vi "Logger.Begin.vi"(8 "error in":errorcluster, 10 "Data in":T1={"BeginTS"=timestamp(0 s since 1904-01-01), "EndTS"=timestamp(0 s since 1904-01-01), "State"=enum."Init", "Status.Work"=enum."-", "Status.Process"=enum."-", "Status.Home"=enum."-", "Status.Wabco"=enum."-", "Status.Client"=enum."-", "BreakReason"=enum."-", "BreakSource"=enum."-", "DoorLock"=FALSE, "Status.Prod"=[], "UserAction"={"Stop"=FALSE, "Pause"=FALSE, "Next"=FALSE}, "UserData"={"GuiMode"=enum."Process", "Test"={"IgnoreResults"=FALSE, "IgnoreImages"=FALSE, "ServiceMode"=FALSE}, "ContinueOrder"=FALSE}, "Error"={"status"=FALSE, "code"=0, "source"=""}, "Code"={"Ready"=FALSE, "DoubleOrder"=FALSE, "OrderDone"=FALSE, "AllowSingleSlot"=FALSE, "CheckDM"=FALSE, "ThresholdA"=0, "ThresholdB"=0, "Plate"=enum."Wabco", "ImgPath"=path "", "Variant"={"State"=enum."Init", "ImgPath"=path "", "WabcoPlate"="", "WabcoProduct"="", "ClientProduct"="", "ClientPlate"="", "TotalQuantity"=0, "OrderQuantity"=0, "Serial"=0, "Wabco"={"LaserJob"="", "AdditionalTxt"="037", "FactoryCode"="", "RevID"=0, "ForkID"=0, "FailuresLimit"=0, "GlobalCnt"=0, "ScannerProgram"=0, "SerialFormat"=enum."6 dig", "CoordA"={"X"=0.0, "Y"=0.0, "Angle"=0.0}, "CoordB"={"X"=0.0, "Y"=0.0, "Angle"=0.0}, "DMCconfig"=0}, "Client"={"LaserJob"="", "AdditionalTxt"="", "FactoryCode"="037", "RevID"=0, "ForkID"=0, "FailuresLimit"=0, "GlobalCnt"=0, "ScannerProgram"=0, "SerialFormat"=enum."6 dig", "CoordA"={"X"=0.0, "Y"=0.0, "Angle"=0.0}, "CoordB"={"X"=0.0, "Y"=0.0, "Angle"=0.0}, "DMCconfig"=0}}}, "Rotations"=0, "ProdIdx"=0, "ProdDone"=[], "PrintedSerials-Wabco"=[], "PrintedSerials-Client"=[], "Counters-Wabco"={"Expected"=0, "Done"=0, "OK"=0, "NOK"=0, "NOKlimit"=0, "Part"=0, "PartOK"=0}, "Counters-Client"={"Expected"=0, "Done"=0, "OK"=0, "NOK"=0, "NOKlimit"=0, "Part"=0, "PartOK"=0}}) -> (0 "error out":errorcluster, 2 "Folder":path, 3 "Refnum out":refnum<k34>)   [LabVIEW 2016]
uses:
  tools/Translator/Translator.Message.ctl
  tools/EventLog/EventLog.EventSource.ctl
  Global/ApplicationGlobal.vi
  tools/EventLog/EventLog.New(single).vi
  Sequence/Sequence.State.ctl
  Gui/MainGui.TestOptions.ctl
  Sequence/Sequence.MainMode.ctl
  Sequence/Sequence.UserData.ctl
  Sequence/Sequence.UserActions.ctl
  Sequence/Sequence.Step.Status.ctl
  Sequence/Sequence.Test.BreakReason.ctl
  Sequence/Sequence.Prod.StatusData.ctl
  Sequence/Sequence.Test.Unload.Status.ctl
  Sequence/Sequence.Slot.StatusData.ctl
  Sequence/Sequence.Test.Status.ctl
  Sequence/Sequence.Code.Sets.ctl
  Sequence/Sequence.Data.ctl
  Logger.Variant.Sets.ctl
  Station/Station.Changeover.State.vi
  Sequence/Sequence.Code.SerialFormat.ctl
  Station/Station.Plate.Properties.ctl
  Drivers/V7310/LowLevel/V7310.Job.Sets.ctl
  Sequence/Sequence.PlateType.ctl
  Sequence/Sequence.Counters.ctl
  Sequence/Sequence.Test.BreakSource.ctl
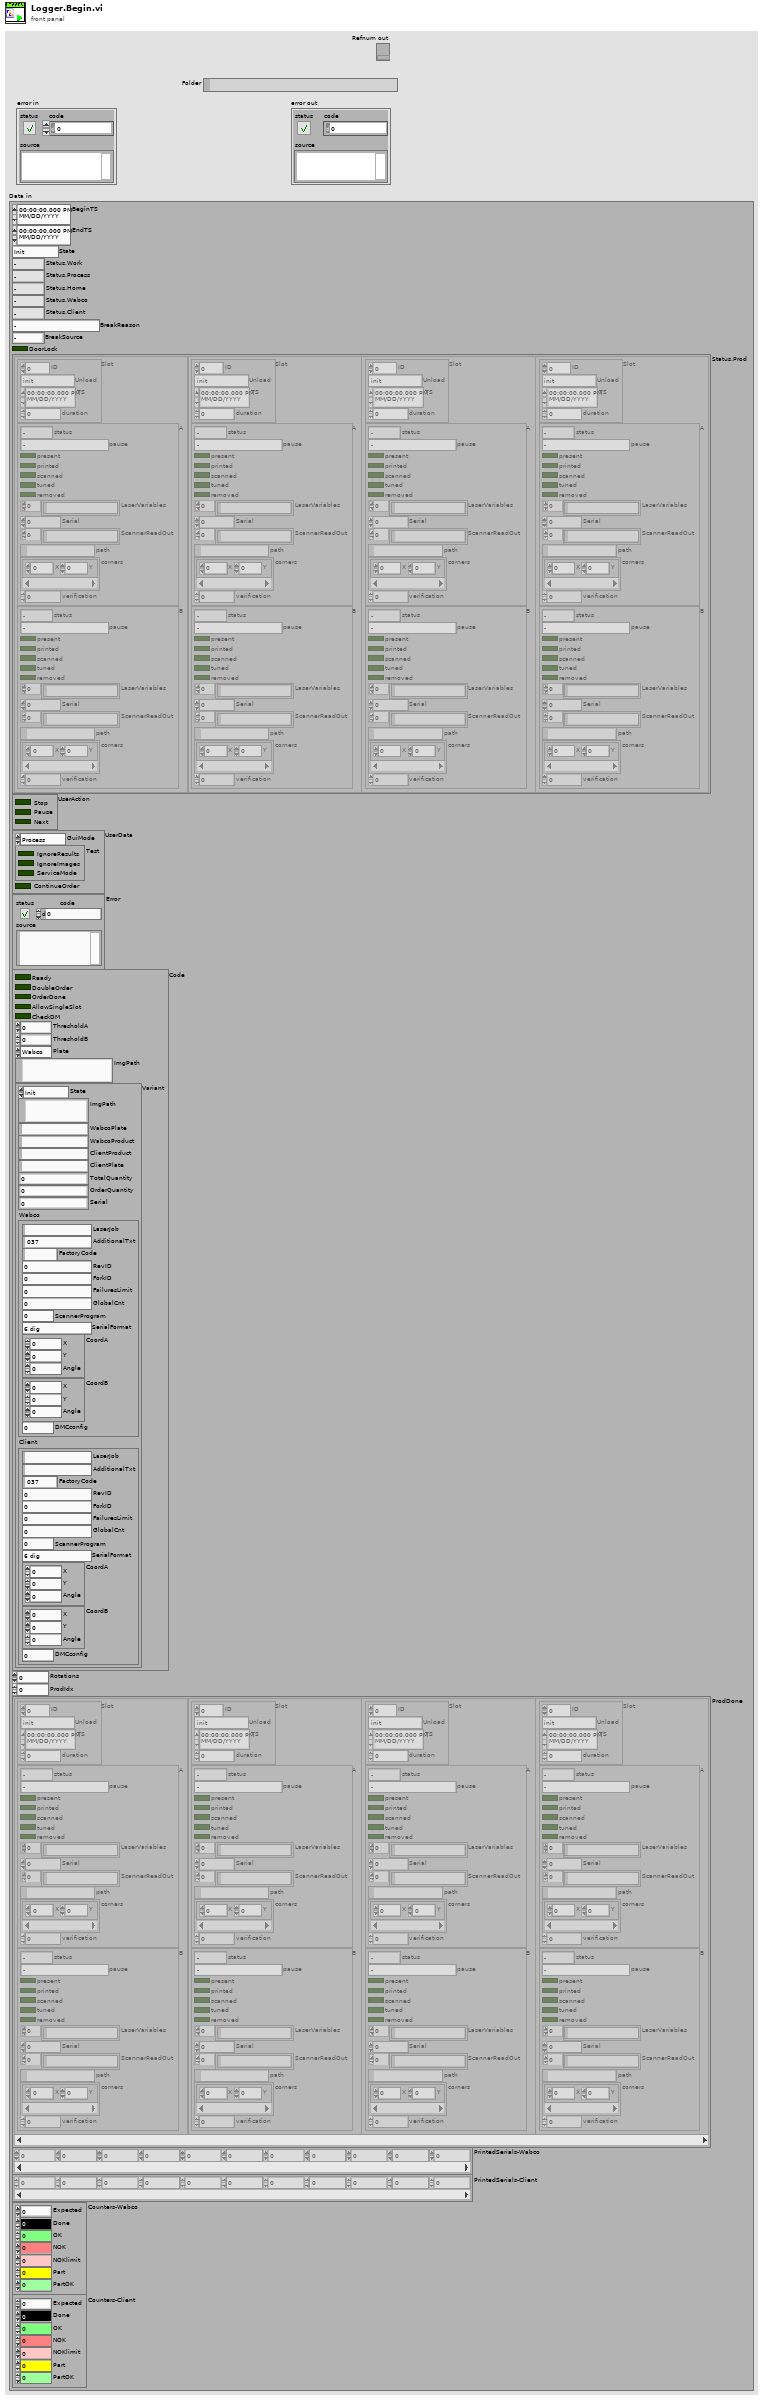
[diagram p1: front panel]
types:
  T1 = typedef "Sequence.Data.ctl" = cluster{"BeginTS":timestamp, "EndTS":timestamp, "State":T2, "Status.Work":T3, "Status.Process":T3, "Status.Home":T3, "Status.Wabco":T3, "Status.Client":T3, "BreakReason":T4, "BreakSource":T5, "DoorLock":bool, "Status.Prod":T6[], "UserAction":T10, "UserData":T11, "Error":errorcluster, "Code":T14, "Rotations":i32, "ProdIdx":i32, "ProdDone":T6[], "PrintedSerials-Wabco":i32[], "PrintedSerials-Client":i32[], "Counters-Wabco":T21, "Counters-Client":T21}
  T2 = typedef "Sequence.State.ctl" = enum16{"Init", "Idle", "Home", "Work", "Run", "Pause"}
  T3 = typedef "Sequence.Step.Status.ctl" = enum16{"-", "Pending", "Running", "Skipped", "Passed", "Failed", "Done", "Error", "Aborted", "Stopped"}
  T4 = typedef "Sequence.Test.BreakReason.ctl" = enum16{"-", "NOK container", "OK container", "Rev empty", "Rev missing", "Rev wrong", "Fork missing", "Fork wrong", "NOK limit", "Unload failure", "Single slot", "Part done", "Err: Prod move work", "Err: Prod move home", "Err: Prod lift work", "Err: Prod lift home", "Err: Prod Arm Work", "Err: Prod Arm NOK", "Err: Prod Arm OK", "Err: Prod NOK suck", "Err: Prod NOK drop", "Err: Prod OK missing", "Err: Prod OK suck", "Err: Prod OK drop"}
  T5 = typedef "Sequence.Test.BreakSource.ctl" = enum16{"-", "A", "B", "A/B"}
  T6 = typedef "Sequence.Test.Status.ctl" = cluster{"Slot":T7, "A":T9, "B":T9}
  T7 = typedef "Sequence.Slot.StatusData.ctl" = cluster{"ID":i32, "Unload":T8, "TS":timestamp, "duration":u32}
  T8 = typedef "Sequence.Test.Unload.Status.ctl" = enum16{"init", "check NOK", "check OK", "wait on NOK", "wait on OK", "wait on Unload", "done"}
  T9 = typedef "Sequence.Prod.StatusData.ctl" = cluster{"status":T3, "pause":T4, "present":bool, "printed":bool, "scanned":bool, "tuned":bool, "removed":bool, "LaserVariables":string[], "Serial":i32, "ScannerReadOut":string[], "path":path, "corners":cluster{"X":i32, "Y":i32}[], "verification":u8}
  T10 = typedef "Sequence.UserActions.ctl" = cluster{"Stop":bool, "Pause":bool, "Next":bool}
  T11 = typedef "Sequence.UserData.ctl" = cluster{"GuiMode":T12, "Test":T13, "ContinueOrder":bool}
  T12 = typedef "Sequence.MainMode.ctl" = enum16{"Process", "Base", "Order", "Manual", "Logs", "Results", "Stats", "DMC Config"}
  T13 = typedef "MainGui.TestOptions.ctl" = cluster{"IgnoreResults":bool, "IgnoreImages":bool, "ServiceMode":bool}
  T14 = typedef "Sequence.Code.Sets.ctl" = cluster{"Ready":bool, "DoubleOrder":bool, "OrderDone":bool, "AllowSingleSlot":bool, "CheckDM":bool, "ThresholdA":u8, "ThresholdB":u8, "Plate":T15, "ImgPath":path, "Variant":T16}
  T15 = typedef "Sequence.PlateType.ctl" = enum16{"Wabco", "Client"}
  T16 = typedef "Logger.Variant.Sets.ctl" = cluster{"State":T17, "ImgPath":path, "WabcoPlate":string, "WabcoProduct":string, "ClientProduct":string, "ClientPlate":string, "TotalQuantity":u16, "OrderQuantity":u16, "Serial":i32, "Wabco":T18, "Client":T18}
  T17 = typedef "Station.Changeover.State.vi" = enum16{"Init", "Scaning", "NOK", "Wait for ack", "Ready"}
  T18 = typedef "Station.Plate.Properties.ctl" = cluster{"LaserJob":string, "AdditionalTxt":string, "FactoryCode":string, "RevID":u8, "ForkID":u8, "FailuresLimit":u16, "GlobalCnt":i32, "ScannerProgram":u8, "SerialFormat":T19, "CoordA":T20, "CoordB":T20, "DMCconfig":i32}
  T19 = typedef "Sequence.Code.SerialFormat.ctl" = enum8{"", "6 dig", "7 dig"}
  T20 = typedef "V7310.Job.Sets.ctl" = cluster{"X":dbl, "Y":dbl, "Angle":dbl}
  T21 = typedef "Sequence.Counters.ctl" = cluster{"Expected":u16, "Done":u16, "OK":u16, "NOK":u16, "NOKlimit":u16, "Part":u16, "PartOK":u16}
  T22 = typedef "EventLog.EventSource.ctl" = enum16{"All", "Gui", "Ref", "File", "Arch", "Seq", "CPX", "DB", "Laser", "Scan.P", "Scan.O"}
  T23 = typedef "Translator.Message.ctl" = enum16{"-", "Event confirmed", "Log out", "Log in", "Shutdown", "Cancel", "Start", "Begin time", "End time", "Duration", "Service Mode", "Ignore Results", "Serial Format", "On", "Off", "OK", "NOK", "NOK %s", "Home", "Work", "Close", "Open", "In progress...", "Missing", "Empty", "Hardware failure", "Initial", "Default", "Total", "Out of range", "Free disk space is below 1GB - contact technician", "Error %d >> %s", "Error %d >> %s >> %s", "Msg %d >> %s", "Laser msg %d %s", "Laser cmd error %s %d", "Laser cmd failed %s", "Laser cmd warning %s", "Laser disconnected", "Laser status %s", "Laser already started", "Laser job unkonwn %s", "Laser job missing %s", "Laser job select failure %s", "Unable to start laser printing (%s)", "Unable to stop laser printing (%s)", "Laser marking aborted", "Laser marking timeout", "Unable to reset Laser Interlock (%s)", "Unable to trigger Laser. Laser not ready (%s)", "Laser job '%s' coordinates not configured", "Starting %s", "Quitting %s", "Configured", "Initializing", "Quitting", "Loading", "Loaded %d results", "Loaded %d events", "Running", "Stopped", "Summary", "Laser", "Do you want to continue?", "Do you want to delete the configuration?", "The configuration is being used by an order. Unable to delete!", "Press confirm button", "Station is not based. Do you want to exit?", "Station requires changeover. Do you want to run the test?", "Test options are not set as default. Do you want to continue?", "Formatting of WabcoNo is disabled. Do you want to continue?", "Product not detected. Do you want to continue?", "Product scan failed. Do you want to continue?", "Calibration", "Log out?", "System", "All", "IDLE", "Translating...%s", "Not found", "Alarm %s", "Run", "Skip", "Abort", "Repeat", "Please wait...", "Database disconnected", "Database disconnected - changeover disabled!", "Login to database successful", "Login to database failed: %d; %s", "Unable to check the product status of reference %d - database disconnected", "Unable to set the product status of reference %d - database disconnected", "Variant file backup %s", "Read variant (%s)", "Result", "Station armed!", "Station requires changeover!", "Select reference number...", "EMERGENCY BUTTON - press Control button", "EMERGENCY DOOR - press Control button", "Resetting Emergency...", "Unable to reset safety circuit - Emergency Button pressed", "Unable to reset safety circuit - Emergency Side Door open", "Station not based", "Station based", "Station not empty", "Station basing...", "No order", "Press Start to begin new order", "Scanning new order", "Order NOK. Correct or scan again", "Order OK. Press Accept", "Order ready", "Revolver incorrect", "Fork incorrect", "Revolver missing", "Revolver empty", "Container missing", "Offline results", "Offline statistics", "Updating statistics %.1f %%", "DMC Configurator", "Door open", "Close the front door", "Press start button", "Done. Open the front door", "Running...", "Running...%.1f %%", "Pause %s", "Pause %s. NOK container missing", "Pause %s. OK container missing", "Pause %s. Revolver empty", "Pause %s. Revolver missing", "Pause %s. Revolver incorrect", "Pause %s. Fork missing", "Pause %s. Fork incorrect", "Pause %s. Too many failures", "Pause %s. Unloading failure", "Pause %s. One slot is not working", "Pause %s. Part order is done. Empty OK container", "Pause %s. Unable to move product to slot", "Pause %s. Unable to move back product pusher", "Pause %s. Unable to lift product", "Pause %s. Unable to move back product lifter", "Pause %s. Unable to move product arm to Work", "Pause %s. Unable to move product arm to NOK", "Pause %s. Unable to move product arm to OK", "Pause %s. Unable to unsuck the NOK product", "Pause %s. Unable to drop the NOK product", "Pause %s. Product OK missing", "Pause %s. Unable to unsuck the OK product", "Pause %s. Unable to drop the OK product", "Stopping...", "File '%s' is missing", "File '%s' is broken", "File '%s' is running", "Log file started (%s)", "Log file ended (%s)", "Log file stopped (%s)", "Log file ignored (%s)", "Log file exported (%s)", "Log file export failed (%s)", "Wrong serial number in log file", "Wrong reference number in log file", "Test steps are missing", "%s = %.3f", "Process param '%s' not found in DB", "Process param '%s' wrong order", "Process param '%s' value %.3f out of limits (%.3f; %.3f)", "Step%d param '%s' not found in DB", "Step%d param '%s' wrong order", "Step%d param '%s' value %.3f out of limits (%.3f; %.3f)", "Step%d EV '%s' not found in DB", "Step%d EV '%s' wrong order", "\"%s\" not found in DB", "\"%s\" wrong order", "\"%s\" value %.3f out of limits (%.3f; %.3f)", "\"%s\" not found in software", "Process init (%s)", "Process started", "Process restarted", "Process run", "Process done", "Process done - remove OK container", "Process aborted", "Process aborted at work", "Process aborted at home", "Process error", "Process error at home", "Process error at work", "Process close", "Process pause", "Process continue", "Process door open", "Process door close", "Process pause at slot %s due to %s", "Select plate from the order to process", "Do you want to start the process?", "Do you want to continue the process?", "There is unfinished order. Do you want to put the new order?", "Product %s %d OK", "Product %s %d NOK", "Unable to unload the slot %s. Product missing in the slot", "Unable to unload the slot %s. Product already in the arm", "Unable to accept the product as OK. Product missing in slot %s", "Unable to accept the product as OK. Product could not drop into the container at slot %s", "Unable to accept the product as NOK. Product could not drop into the container at slot %s", "Scan failed. Error %s", "Scan failed. Scanner disconnected", "Scan failed. Wrong Wabco number %d, limit (%d,%d)", "Scan failed. Wrong serial number %d, limit (%d,%d)", "Scan failed. Wrong date %d, limit (%d,%d)", "Scan failed. Wrong product wabco number %d (expected %d)", "Scan failed. Wrong product serial number %d (expected > 0)", "Scan OK %s", "Scan failed. Unable to determine table position (%s)", "Scan failed. Timeout", "Tune failed. Scanner disconnected", "Tune failed. Timeout", "%s = %d", "%s = %d->%d", "Unable to set %s = %.2f - Air Pressure Inside off", "Unable to set digital output '%s' = %d", "Unable to activate air pressure inside - timeout", "Unable to activate air pressure inside - aborted", "Unable to switch on Air Main Valve - Air Pressure Inlet off", "Unable to switch on Air Main Valve - Door open", "Unable to switch off Air Main Valve - timeout", "Unable to switch off Air Main Valve - aborted", "Unable to rotate Table - timeout", "Unable to rotate Table - aborted", "Unable to rotate Table - Product Move not in Home position", "Unable to rotate Table - Air Pressure Inside off", "Unable to rotate Table - Product Lift A not in Home position", "Unable to rotate Table - Product Lift B not in Home position", "Unable to rotate Table - unlock before movement timeout", "Unable to rotate Table - lock after movement timeout", "Unable to move Table Lock to %s position - timeout", "Unable to move Table Lock to %s position - aborted", "Unable to move Table Lock to %s position - Air Pressure Inside off", "Unable to move Table Lock to %s position - Table not in position", "Unable to move Product Lift A to %s position - timeout", "Unable to move Product Lift B to %s position - timeout", "Unable to move Product Lift A to %s position - aborted", "Unable to move Product Lift B to %s position - aborted", "Unable to move Product Lift A to %s position - Air Pressure Inside off", "Unable to move Product Lift B to %s position - Air Pressure Inside off", "Unable to move Product Lift A to %s position - Table not locked", "Unable to move Product Lift B to %s position - Table not locked", "Unable to move Product Lift A to %s position - Product Arm not in Work position", "Unable to move Product Lift B to %s position - Product Arm not in Work position", "Unable to set Product Suction Gripper %s to %s - timeout", "Unable to set Product Suction Gripper %s to %s - aborted", "Unable to set Product Suction Gripper %s to %s - Air Pressure Inside off", "Unable to set Product Suction Gripper %s to %s - Table slot unkown", "Unable to move Product Arm to %s position - timeout", "Unable to move Product Arm to %s position - aborted", "Unable to move Product Arm to %s position - Air Pressure Inside off", "Unable to move Product Arm to %s position - Product Lift A not in Home position", "Unable to move Product Arm to %s position - Product Lift B not in Home position", "Unable to move Product to %s position - timeout", "Unable to move Product to %s position - aborted", "Unable to move Product to %s position - Air Pressure Inside off", "Unable to move Product to %s position - Table not in position"}
  T24 = enum16{"open", "open or create", "create or replace", "create", "open (read-only)"}
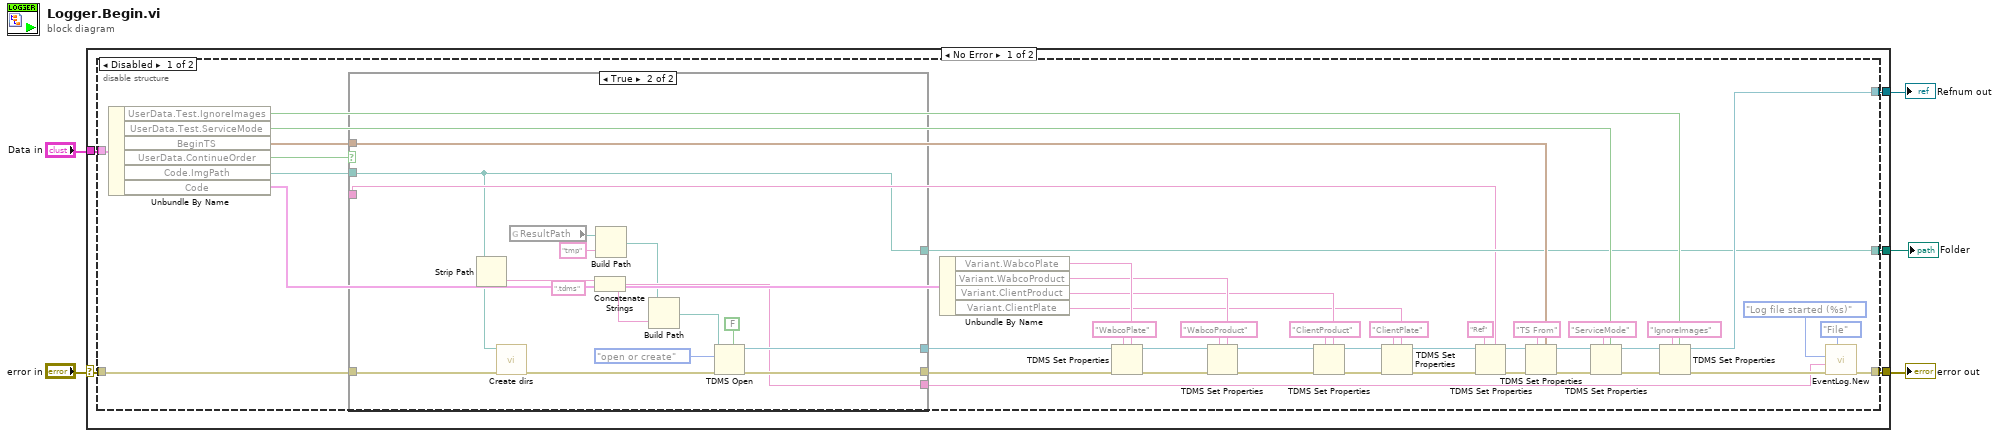
[diagram p0: block diagram]
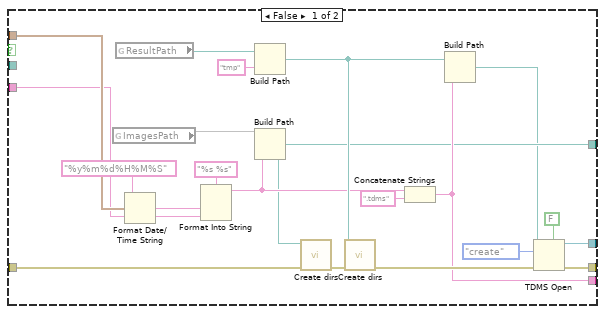
[diagram p2: hidden frame]
diagram:
  n1 = case shown="No Error" "error in" {
    selector: "error in" -> [w7 w90]
    tunnel: [w8 _] -> w5
    tunnel: [w10 w90] -> w4
    tunnel: "Data in" -> [w9 _]
    tunnel: [w6 _] -> w1
    frame No Error {
      n2 = disable-structure shown="Disabled" {
        disable-tunnel: [w54 _] -> w10
        disable-tunnel: w9 -> [w53 _]
        disable-tunnel: [w37 _] -> w8
        disable-tunnel: w7 -> [w34 _]
        disable-tunnel: [w33 _] -> w6
        frame Disabled {
          n3 = Unbundle By Name(w53) -> ("UserData.Test.IgnoreImages"=w40:bool, "UserData.Test.ServiceMode"=w41:bool, "BeginTS"=w36:timestamp, "UserData.ContinueOrder"=w32:bool, "Code.ImgPath"=w31:path, "Code"=w29:T14)
          n4 = case shown="True" w32 {
            tunnel: [w72 w84] -> w18
            tunnel: [w71 w85] -> w15
            tunnel: w36 -> [w68 _]
            tunnel: [w62 w79] -> w35
            tunnel: w34 -> [w61 w87]
            tunnel: [w58 w76] -> w33
            tunnel: w31 -> [_ w76]
            tunnel: [w57 _] -> w30
            frame False {
              n5 = global read "ApplicationGlobal.vi" "ImagesPath"() -> (w64)
              n6 = global read "ApplicationGlobal.vi" "ResultPath"() -> (w56:path)
              n7 = Format Date/Time String(time format string (%c)="%y%m%d%H%M%S", seconds (now)=w68) -> (date/time string=w65:string)  [unwired: 1 in]
              n8 = Format Into String(format string="%s %s", w65, w57) -> (resulting string=w59:string)  [unwired: 2 in, 1 out]
              n9 = Build Path(base path=w56, name or relative path="tmp") -> (appended path=w67:path)
              n10 = Build Path(base path=w64, name or relative path=w59) -> (appended path=w58:path)
              n11 = call "Create dirs.vi"("error in (no error)"=w61, "deepest dir"=w58) -> ("error"=w60:errorcluster)  [unwired: 9 in]
              n12 = call "Create dirs.vi"("error in (no error)"=w60, "deepest dir"=w67) -> ("error"=w74:errorcluster)  [unwired: 9 in]
              n13 = Concatenate Strings(w59, ".tdms" ("string")) -> (w62:string)
              n14 = Build Path(base path=w67, name or relative path=w62) -> (appended path=w55:path)
              n15 = TDMS Open(5:FALSE ("create index file? (T)"), 8:w74, 10:T24."create" ("operation (0:open)"), 11:w55) -> (0:w71:errorcluster, 3:w72:refnum<k34>)  [unwired: 3 in]
            }
            frame True {
              n16 = Strip Path(path=w76) -> (name=w82:string)  [unwired: 1 out]
              n17 = call "Create dirs.vi"("error in (no error)"=w87, "deepest dir"=w76) -> ("error"=w86:errorcluster)  [unwired: 9 in]
              n18 = global read "ApplicationGlobal.vi" "ResultPath"() -> (w81:path)
              n19 = Concatenate Strings(w82, ".tdms" ("string")) -> (w79:string)
              n20 = Build Path(base path=w81, name or relative path="tmp") -> (appended path=w78:path)
              n21 = Build Path(base path=w78, name or relative path=w79) -> (appended path=w77:path)
              n22 = TDMS Open(5:FALSE ("create index file? (T)"), 8:w86, 10:T24."open or create" ("operation (0:open)"), 11:w77) -> (0:w85:errorcluster, 3:w84:refnum<k34>)  [unwired: 3 in]
            }
          }
          n23 = Unbundle By Name(w29) -> ("Variant.WabcoPlate"=w14:string, "Variant.WabcoProduct"=w13:string, "Variant.ClientProduct"=w12:string, "Variant.ClientPlate"=w11:string)
          n24 = TDMS Set Properties(5:w14, 7:"WabcoPlate", 8:w15, 11:w18) -> (0:w20:errorcluster, 3:w21:refnum<k34>)  [unwired: 2 in, 2 out]
          n25 = TDMS Set Properties(5:w13, 7:"WabcoProduct", 8:w20, 11:w21) -> (0:w25:errorcluster, 3:w26:refnum<k34>)  [unwired: 2 in, 2 out]
          n26 = TDMS Set Properties(5:w12, 7:"ClientProduct", 8:w25, 11:w26) -> (0:w28:errorcluster, 3:w24:refnum<k34>)  [unwired: 2 in, 2 out]
          n27 = TDMS Set Properties(5:w11, 7:"ClientPlate", 8:w28, 11:w24) -> (0:w16:errorcluster, 3:w17:refnum<k34>)  [unwired: 2 in, 2 out]
          n28 = TDMS Set Properties(5:w30, 7:"Ref", 8:w16, 11:w17) -> (0:w49:errorcluster, 3:w48:refnum<k34>)  [unwired: 2 in, 2 out]
          n29 = TDMS Set Properties(5:w36, 7:"TS From", 8:w49, 11:w48) -> (0:w44:errorcluster, 3:w43:refnum<k34>)  [unwired: 2 in, 2 out]
          n30 = TDMS Set Properties(5:w41, 7:"ServiceMode", 8:w44, 11:w43) -> (0:w38:errorcluster, 3:w45:refnum<k34>)  [unwired: 2 in, 2 out]
          n31 = TDMS Set Properties(5:w40, 7:"IgnoreImages", 8:w38, 11:w45) -> (0:w42:errorcluster, 3:w37:refnum<k34>)  [unwired: 2 in, 2 out]
          n32 = call-poly "EventLog.New.vi"("Source (All)"=EventLog.EventSource."File" ("Source (App)"), "error in (no error)"=w42, "Arg"=w35, "Message (-)"=Translator.Message."Log file started (%s)") -> ("error out"=w54:errorcluster)  [unwired: 6 in, 1 out]
        }
        frame Enabled {
        }
      }
    }
    frame Error {
    }
  }
  "Refnum out" <- w5
  "error out" <- w4
  "Folder" <- w1
